vi "Control Globals.vi"() -> ()   [LabVIEW 2017]
panel:
  in  "Lidar Data Queue":refnum<queue>
  out "Slam Works":bool
  in  "Shared Library Path":path=path "/home/admin/lib/libslam.so"
  out "Lidar Works":bool
  out "Gyro Works":bool
  in  "Pose":cluster{"X":dbl, "Y":dbl, "R":dbl}
  in  "Pose Update Queue":refnum<queue>
  out "Stopping":bool
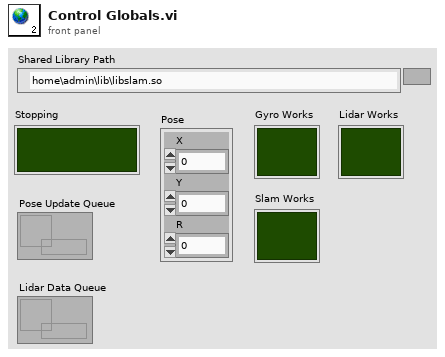
[diagram p1: front panel]
diagram:
